vi "auto.vi"(8 "error in (no error)":errorcluster) -> (0 "error out":errorcluster)   [LabVIEW 2014]
uses:
  <vilib>/Rock Robotics/WPI/RobotDrive/WPI_RobotDriveMecanumDrive_Cartesian.vi
  <vilib>/Rock Robotics/WPI/Solenoid/WPI_SolenoidSetEnum.vi
  <vilib>/Rock Robotics/WPI/Solenoid/WPI_SolenoidValue.ctl
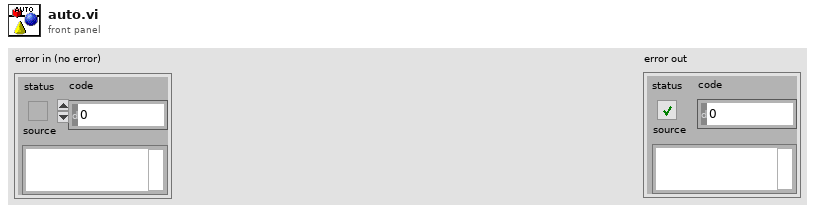
[diagram p1: front panel]
types:
  T1 = typedef "WPI_SolenoidDevRef.ctl" = cluster{"DevStatus":errorcluster, "Pneumatics Control Module":u8, "Forward Solenoid Channel":T2, "Reverse Solenoid Channel":T2}
  T2 = typedef "WPI_SolenoidChannel.ctl" = enum8{"Solenoid 0", "Solenoid 1", "Solenoid 2", "Solenoid 3", "Solenoid 4", "Solenoid 5", "Solenoid 6", "Solenoid 7", "Invalid"}
  T3 = typedef "WPI_RobotDriveDevRef.ctl" = cluster{"DevStatus":errorcluster, "Motors[]":T4[], "Square Inputs":bool, "Max Output":dbl}
  T4 = typedef "WPI_MotorControlDeviceRef.ctl" = cluster{"DeviceStatus":errorcluster, "Type":T5, "PWM":cluster{"Controller":T6, "PWM Channel":T7, "DeadBand":T8}, "CAN":cluster{"Device Number":u8, "Control Mode":T9, "Semaphore":T10, "Max Vout":dbl, "TalonSRX Control Mode":T11}, "Invert":bool, "TransformRef":T12, "InvTransformRef":T12}
  T5 = typedef "WPI_MotorControlType.ctl" = enum16{"PWM", "CAN", "CANTalonSRX"}
  T6 = typedef "FPGA_TypedefDigitalModule.ctl" = enum16{"Controller 1"}
  T7 = typedef "FPGA_DIOPWMChannel.ctl" = enum8{"PWM 0", "PWM 1", "PWM 2", "PWM 3", "PWM 4", "PWM 5", "PWM 6", "PWM 7", "PWM 8", "PWM 9", "PWM MXP 0", "PWM MXP 1", "PWM MXP 2", "PWM MXP 3", "PWM MXP 4", "PWM MXP 5", "PWM MXP 6", "PWM MXP 7", "PWM MXP 8", "PWM MXP 9", "Invalid"}
  T8 = typedef "WPI_PWMDeadband.ctl" = cluster{"Name":string, "maxPositivePwm":i32, "minPositivePwm":i32, "centerPwm":i32, "maxNegativePwm":i32, "minNegativePwm":i32, "angularRange":u16}
  T9 = typedef "WPI_CANJaguar_ControlMode.ctl" = enum8{"Percent VBus", "Current", "Speed", "Position", "Voltage"}
  T10 = typedef "Semaphore RefNum" = refnum<k1>
  T11 = typedef "WPI_CANTalonSRX_APIControlMode.ctl" = enum8{"Percent VBus", "Speed", "Position", "Slave", "Unchanged / Invalid"}
  T12 = typedef "WPI_PWMTransform_ConPane.ctl" = refnum<vi>
  T13 = typedef "WPI_SolenoidValue.ctl" = enum16{"Off", "On", "Forward", "Reverse"}
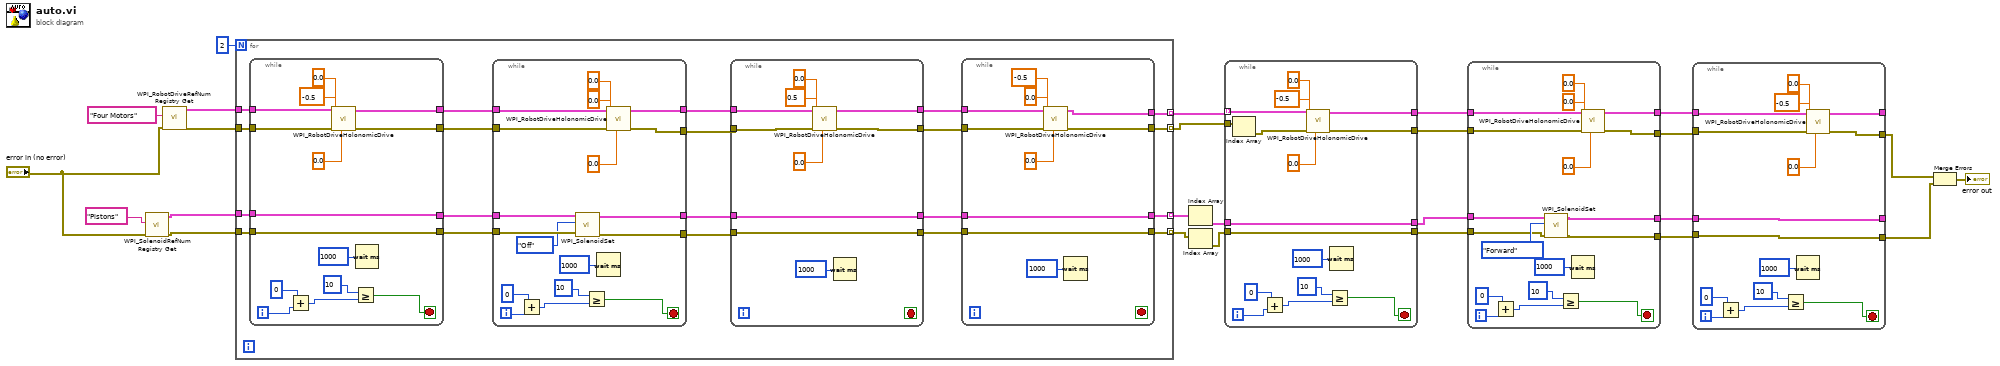
[diagram p0: block diagram]
diagram:
  n1 = call <vilib>:"WPI_SolenoidRefNum Registry Get.vi"("error in (no error)"="error in (no error)", "refnum name"="Pistons") -> ("error out"=w14:errorcluster, "SolenoidDevRef"=w9:T1)  [unwired: 8 in]
  n2 = call <vilib>:"WPI_RobotDriveRefNum Registry Get.vi"("error in (no error)"="error in (no error)", "refnum name"="Four Motors") -> ("error out"=w23:errorcluster, "RobotDriveDevRef"=w24:T3)  [unwired: 8 in]
  n3 = for {
    N: 2 -> [_]
    tunnel: w24 -> [w45]
    tunnel: w9 -> [w44]
    tunnel: w14 -> [w42]
    tunnel: w23 -> [w38]
    tunnel: [w31] -> w19 mode=indexing
    tunnel: [w30] -> w7 mode=indexing
    tunnel: [w27] -> w6 mode=indexing
    tunnel: [w26] -> w1 mode=indexing
    n4 = while {
      tunnel: w45 -> [w98]
      tunnel: [w93] -> w43
      tunnel: w44 -> [w93]
      tunnel: w42 -> [w92]
      tunnel: [w92] -> w41
      tunnel: [w91] -> w40
      tunnel: [w90] -> w39
      tunnel: w38 -> [w89]
      i -> [w86]
      stop <- w84 stop-if-true
      n5 = Add(x=0, y=w86) -> (x+y=w85:i32)
      n6 = call-poly <vilib>:"WPI_RobotDriveHolonomicDrive.vi"("Rotation"=0.0, "error in (no error)"=w89, "Y"=0.0, "X"=-0.5, "RobotDriveDevRef"=w98) -> ("error out"=w90:errorcluster, "RobotDriveDevRef"=w91:T3)  [unwired: 4 in, 1 out]
      n7 = Greater Or Equal?(x=10, y=w85) -> (x >= y?=w84:bool)
      n8 = Wait (ms)(milliseconds to wait=u32 1000) -> ()  [unwired: 1 out]
    }
    n9 = while {
      tunnel: w43 -> [w70]
      tunnel: w41 -> [w69]
      tunnel: w40 -> [w79]
      tunnel: w39 -> [w78]
      tunnel: [w77] -> w37
      tunnel: [w76] -> w36
      tunnel: [w68] -> w35
      tunnel: [w66] -> w29
      i -> [w75]
      stop <- w71 stop-if-true
      n10 = Add(x=0, y=w75) -> (x+y=w73:i32)
      n11 = call-poly <vilib>:"WPI_SolenoidSet.vi"("error in (no error)"=w69, "Value"=WPI_SolenoidValue."Off", "SolenoidDevRef"=w70) -> ("error out"=w68:errorcluster, "SolenoidDevRef"=w66:T1)  [unwired: 7 in]
      n12 = Greater Or Equal?(x=10, y=w73) -> (x >= y?=w71:bool)
      n13 = Wait (ms)(milliseconds to wait=u32 1000) -> ()  [unwired: 1 out]
      n14 = call-poly <vilib>:"WPI_RobotDriveHolonomicDrive.vi"("Rotation"=0.0, "error in (no error)"=w78, "Y"=0.0, "X"=0.0, "RobotDriveDevRef"=w79) -> ("error out"=w76:errorcluster, "RobotDriveDevRef"=w77:T3)  [unwired: 4 in, 1 out]
    }
    n15 = while {
      tunnel: w37 -> [w65]
      tunnel: w35 -> [w60]
      tunnel: [w60] -> w32
      tunnel: [w59] -> w34
      tunnel: [w58] -> w33
      tunnel: w36 -> [w57]
      tunnel: [w56] -> w28
      tunnel: w29 -> [w56]
      stop <- _ stop-if-true
      n16 = call-poly <vilib>:"WPI_RobotDriveHolonomicDrive.vi"("Rotation"=0.0, "error in (no error)"=w57, "Y"=0.0, "X"=0.5, "RobotDriveDevRef"=w65) -> ("error out"=w58:errorcluster, "RobotDriveDevRef"=w59:T3)  [unwired: 4 in, 1 out]
      n17 = Wait (ms)(milliseconds to wait=u32 1000) -> ()  [unwired: 1 out]
    }
    n18 = while {
      tunnel: w34 -> [w55]
      tunnel: w32 -> [w50]
      tunnel: [w50] -> w26
      tunnel: [w49] -> w31
      tunnel: [w48] -> w30
      tunnel: w33 -> [w47]
      tunnel: [w46] -> w27
      tunnel: w28 -> [w46]
      stop <- _ stop-if-true
      n19 = call-poly <vilib>:"WPI_RobotDriveHolonomicDrive.vi"("Rotation"=0.0, "error in (no error)"=w47, "Y"=-0.5, "X"=0.0, "RobotDriveDevRef"=w55) -> ("error out"=w48:errorcluster, "RobotDriveDevRef"=w49:T3)  [unwired: 4 in, 1 out]
      n20 = Wait (ms)(milliseconds to wait=u32 1000) -> ()  [unwired: 1 out]
    }
  }
  n21 = Index Array(array=w6) -> (element=w5:T1)  [unwired: 1 in]
  n22 = Index Array(array=w1) -> (element=w2:errorcluster)  [unwired: 1 in]
  n23 = while {
    tunnel: w19 -> [w114] mode=indexing
    tunnel: [w109] -> w21
    tunnel: [w108] -> w20
    tunnel: w7 -> [w102]
    tunnel: w5 -> [w100]
    tunnel: [w100] -> w4
    tunnel: [w99] -> w3
    tunnel: w2 -> [w99]
    i -> [w105]
    stop <- w103 stop-if-true
    n24 = Index Array(array=w102) -> (element=w101:errorcluster)  [unwired: 1 in]
    n25 = Add(x=0, y=w105) -> (x+y=w104:i32)
    n26 = call-poly <vilib>:"WPI_RobotDriveHolonomicDrive.vi"("Rotation"=0.0, "error in (no error)"=w101, "Y"=0.0, "X"=-0.5, "RobotDriveDevRef"=w114) -> ("error out"=w108:errorcluster, "RobotDriveDevRef"=w109:T3)  [unwired: 4 in, 1 out]
    n27 = Greater Or Equal?(x=10, y=w104) -> (x >= y?=w103:bool)
    n28 = Wait (ms)(milliseconds to wait=u32 1000) -> ()  [unwired: 1 out]
  }
  n29 = while {
    tunnel: w21 -> [w128]
    tunnel: w20 -> [w127]
    tunnel: [w126] -> w18
    tunnel: [w125] -> w17
    tunnel: [w119] -> w16
    tunnel: [w118] -> w15
    tunnel: w4 -> [w116]
    tunnel: w3 -> [w115]
    i -> [w124]
    stop <- w120 stop-if-true
    n30 = Add(x=0, y=w124) -> (x+y=w122:i32)
    n31 = call-poly <vilib>:"WPI_SolenoidSet.vi"("error in (no error)"=w115, "Value"=WPI_SolenoidValue."Forward", "SolenoidDevRef"=w116) -> ("error out"=w118:errorcluster, "SolenoidDevRef"=w119:T1)  [unwired: 7 in]
    n32 = Greater Or Equal?(x=10, y=w122) -> (x >= y?=w120:bool)
    n33 = Wait (ms)(milliseconds to wait=u32 1000) -> ()  [unwired: 1 out]
    n34 = call-poly <vilib>:"WPI_RobotDriveHolonomicDrive.vi"("Rotation"=0.0, "error in (no error)"=w127, "Y"=0.0, "X"=0.0, "RobotDriveDevRef"=w128) -> ("error out"=w125:errorcluster, "RobotDriveDevRef"=w126:T3)  [unwired: 4 in, 1 out]
  }
  n35 = while {
    tunnel: w16 -> [w133]
    tunnel: w15 -> [w134]
    tunnel: w18 -> [w143]
    tunnel: w17 -> [w142]
    tunnel: [w141] -> _
    tunnel: [w140] -> w12
    tunnel: [w133] -> _
    tunnel: [w134] -> w11
    i -> [w139]
    stop <- w135 stop-if-true
    n36 = Add(x=0, y=w139) -> (x+y=w137:i32)
    n37 = Greater Or Equal?(x=10, y=w137) -> (x >= y?=w135:bool)
    n38 = Wait (ms)(milliseconds to wait=u32 1000) -> ()  [unwired: 1 out]
    n39 = call-poly <vilib>:"WPI_RobotDriveHolonomicDrive.vi"("Rotation"=0.0, "error in (no error)"=w142, "Y"=0.0, "X"=-0.5, "RobotDriveDevRef"=w143) -> ("error out"=w140:errorcluster, "RobotDriveDevRef"=w141:T3)  [unwired: 4 in, 1 out]
  }
  n40 = Merge Errors(w12, w11) -> (→"error out":errorcluster)
